vi "Template Update.vi"(8 "error in (no error)":errorcluster, 9 "Parameters (empty)":T2, 10 "Template Record":T1, 11 "Connection Refnum":T3) -> (0 "error out":errorcluster, 2 "New Template Record":T1, 3 "Connection Refnum":T3)   [LabVIEW 2011]
uses:
  Template Record.ctl
  SI.LIB/ODBC/SQL Controls/Connection Refnum.ctl
  Addons/internet/utils/keyedarr.llb/Keyed Array.ctl
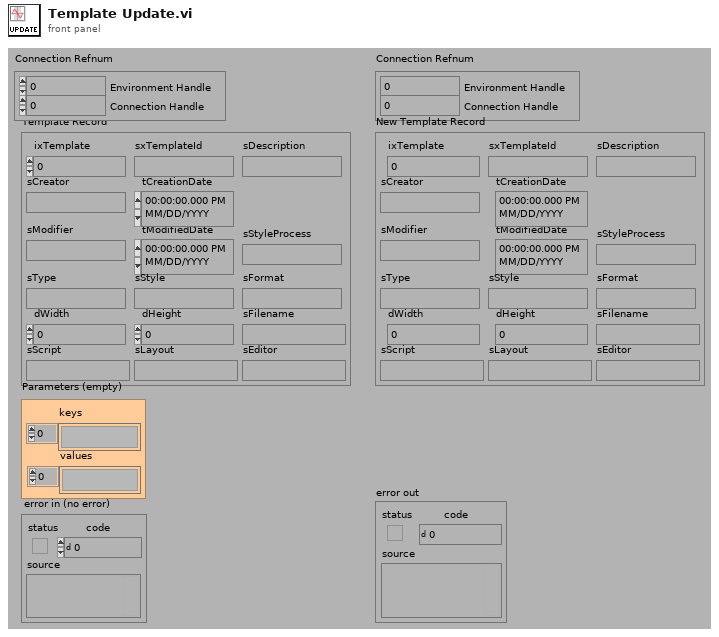
[diagram p1: front panel]
types:
  T1 = typedef "Template Record.ctl" = cluster{"ixTemplate":i32, "sxTemplateId":string, "sDescription":string, "sCreator":string, "tCreationDate":timestamp, "sModifier":string, "tModifiedDate":timestamp, "sType":string, "sStyle":string, "sFormat":string, "dWidth":dbl, "dHeight":dbl, "sFilename":string, "sScript":string, "sLayout":string, "sEditor":string, "sStyleProcess":string}
  T2 = typedef "Keyed Array.ctl" = cluster{"keys":string[], "values":string[]}
  T3 = typedef "Connection Refnum.ctl" = cluster{"Environment Handle":i32, "Connection Handle":i32}
  T4 = typedef "Statement Refnum.ctl" = cluster{"Statement Handle":i32, "Parameter Number":u16}
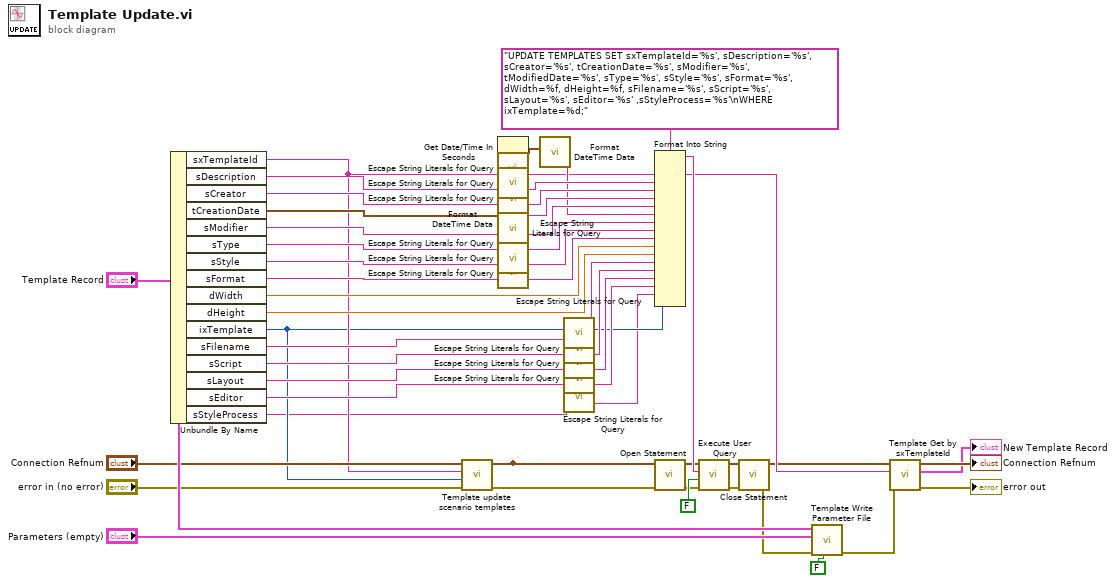
[diagram p0: block diagram]
diagram:
  n1 = Unbundle By Name("Template Record") -> ("sxTemplateId"=w4:string, "sDescription"=w35:string, "sCreator"=w34:string, "tCreationDate"=w33:timestamp, "sModifier"=w31:string, "sType"=w29:string, "sStyle"=w28:string, "sFormat"=w27:string, "dWidth"=w23:dbl, "dHeight"=w22:dbl, "ixTemplate"=w3:i32, "sFilename"=w37:string, "sScript"=w40:string, "sLayout"=w39:string, "sEditor"=w38:string, "sStyleProcess"=w2:string)
  n2 = call "Template update scenario templates.vi"("error in (no error)"="error in (no error)", "ixTemplate (0)"=w3, "new name"=w4, "Connection Refnum"="Connection Refnum") -> ("error out"=w5:errorcluster, "Connection Refnum"=w6:T3)  [unwired: 6 out]
  n3 = Get Date/Time In Seconds() -> (seconds since 1Jan1904=w36:timestamp)
  n4 = call "Escape String Literals for Query.vi"("String"=w4) -> ("escaped String"=w15:string)  [unwired: 1 in, 13 out]
  n5 = call "Escape String Literals for Query.vi"("String"=w35) -> ("escaped String"=w41:string)  [unwired: 1 in, 13 out]
  n6 = call "Escape String Literals for Query.vi"("String"=w34) -> ("escaped String"=w43:string)  [unwired: 1 in, 13 out]
  n7 = call "Format DateTime Data.vi"("Timestamp in"=w33) -> ("UTC DB String out"=w32:string)  [unwired: 10 out]
  n8 = call "Escape String Literals for Query.vi"("String"=w31) -> ("escaped String"=w42:string)  [unwired: 1 in, 13 out]
  n9 = call "Escape String Literals for Query.vi"("String"=w29) -> ("escaped String"=w26:string)  [unwired: 1 in, 13 out]
  n10 = call "Escape String Literals for Query.vi"("String"=w28) -> ("escaped String"=w25:string)  [unwired: 1 in, 13 out]
  n11 = call "Escape String Literals for Query.vi"("String"=w27) -> ("escaped String"=w24:string)  [unwired: 1 in, 13 out]
  n12 = call "Format DateTime Data.vi"("Timestamp in"=w36) -> ("UTC DB String out"=w30:string)  [unwired: 10 out]
  n13 = call "Escape String Literals for Query.vi"("String"=w37) -> ("escaped String"=w21:string)  [unwired: 1 in, 13 out]
  n14 = call "Escape String Literals for Query.vi"("String"=w40) -> ("escaped String"=w20:string)  [unwired: 1 in, 13 out]
  n15 = call "Escape String Literals for Query.vi"("String"=w39) -> ("escaped String"=w19:string)  [unwired: 1 in, 13 out]
  n16 = call "Escape String Literals for Query.vi"("String"=w38) -> ("escaped String"=w18:string)  [unwired: 1 in, 13 out]
  n17 = call "Escape String Literals for Query.vi"("String"=w2) -> ("escaped String"=w1:string)  [unwired: 1 in, 13 out]
  n18 = Format Into String(format string="UPDATE TEMPLATES SET sxTemplateId='%s', sDescription='%s', sCreator='%s', tCreationDate='%s', sModifier='%s', tModifiedDate='%s', sType='%s', sStyle='%s', sFormat='%s', dWidth=%f, dHeight=%f, sFilename='%s', sScript='%s', sLayout='%s', sEditor='%s' ,sStyleProcess='%s'\nWHERE ixTemplate=%d;" ("User Query"), w15, w41, w43, w32, w42, w30, w26, w25, w24, w23, w22, w21, w20, w19, w18, w1, w3) -> (resulting string=w46:string)  [unwired: 2 in, 1 out]
  n19 = call "Open Statement.vi"("error in (no error)"=w5, "Connection Refnum"=w6) -> ("error out"=w45:errorcluster, "Statement Refnum"=w44:T4)  [unwired: 4 out]
  n20 = call "Execute User Query.vi"("error in (no error)"=w45, "Return Data? (f)"=FALSE, "User Query"=w46, "Statement Refnum"=w44) -> ("error out"=w49:errorcluster, "Statement Refnum"=w48:T4)  [unwired: 2 out]
  n21 = call "Close Statement.vi"("error in (no error)"=w49, "Statement Refnum"=w48) -> ("error out"=w10:errorcluster)  [unwired: 5 out]
  n22 = call "Template Write Parameter File.vi"("Export?"=FALSE ("Load Content for export?"), "error in (no error)"=w10, "Parameters (empty)"="Parameters (empty)", "Template Record"="Template Record") -> ("error out"=w9:errorcluster)  [unwired: 2 in, 5 out]
  n23 = call "Template Get by sxTemplateId.vi"("error in (no error)"=w9, "sxTemplateId (\"\")"=w15, "Connection Refnum"=w6) -> ("error out"=→"error out":errorcluster, "Template Record"=→"New Template Record":T1, "Connection Refnum"=→"Connection Refnum":T3)  [unwired: 6 out]
